vi "Pll_Lock_Detect.vi"(0 "COMPORT":refnum<visa-resource-name>="COM6", 11 "error in (no error)":errorcluster, 12 "CLK_USAGE":u16(ring) items=["EXT CLK", "INT CLK"], 13 "Open Serial":bool, 14 "Close Serial":bool) -> (3 "PllSuccess?(T)":bool, 15 "error out":errorcluster)   [LabVIEW 2018]
panel:
  in  "Command ( ; seperation)":string="pmb 0x69 wr 0xff 00;pmb 0x69 wr 0x07 rd 1"
  out "string":string="caladc\r\n>\ncaladc -r\r\ncaladc delay: 0x00004333\r\n>\r\n"
  out "count?(t)":bool
  out "result(i32)":i32
  out "Reg 0x07":string
  out "Readback Success?(t)":bool
  # "THIS VI IS DESIGNED TO DETECT THE HOLDOVER/LOCK STATE OF  CLOCK"
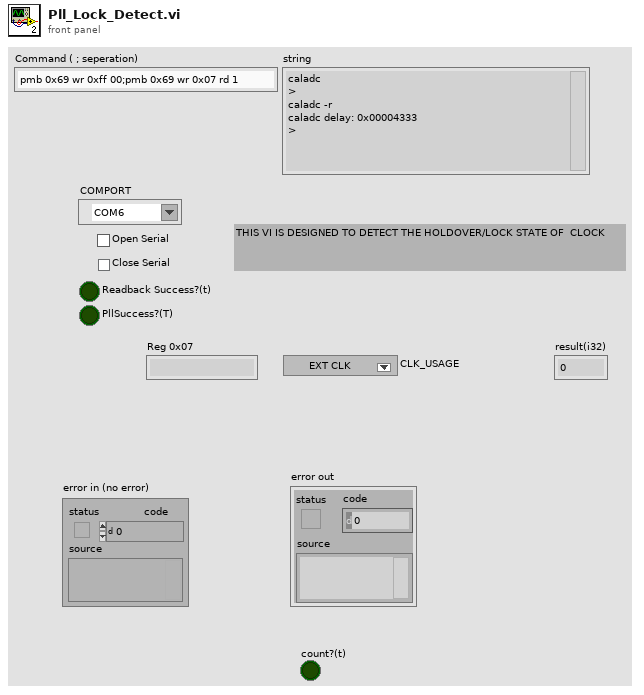
[diagram p1: front panel]
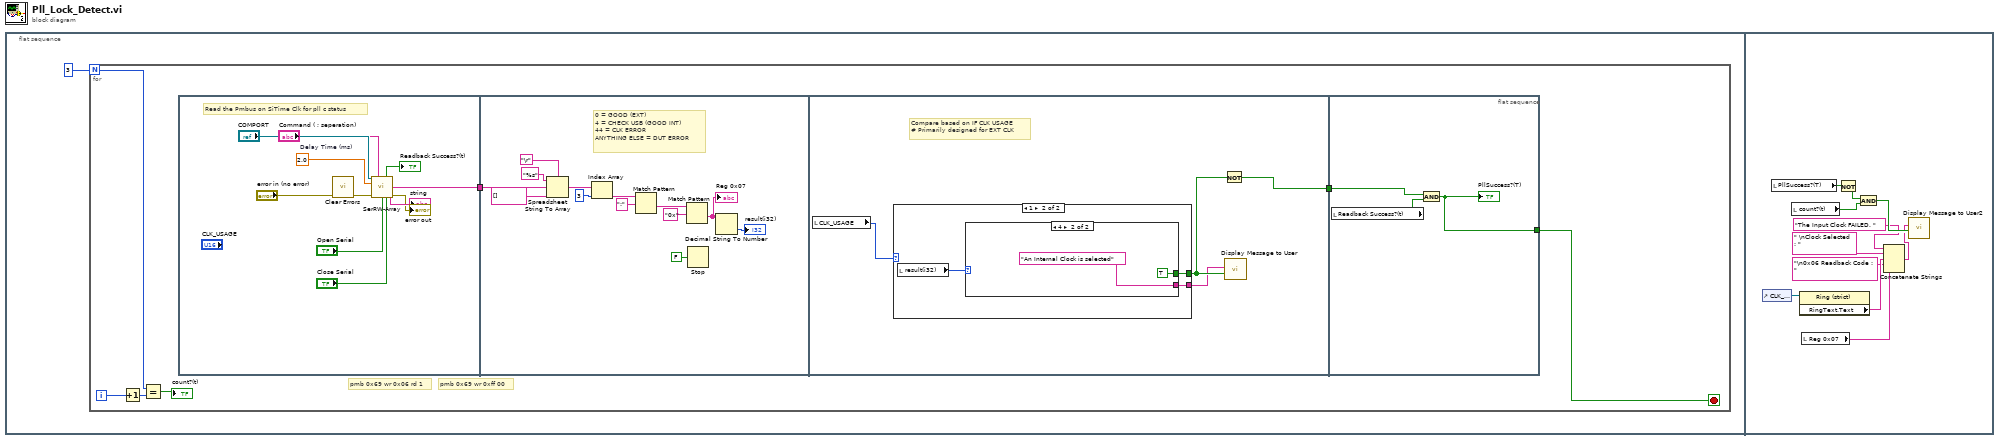
[diagram p0: block diagram]
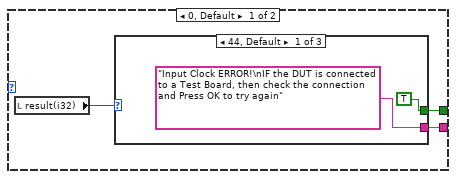
[diagram p2: hidden frame]
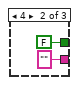
[diagram p3: hidden frame]
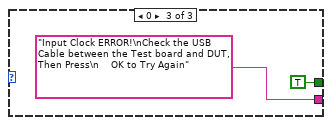
[diagram p4: hidden frame]
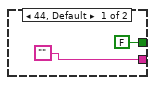
[diagram p5: hidden frame]
diagram:
  n1 = flat-sequence {
    frame #0 {
      n2 = for {
        N: 3 -> [w5]
        i -> [w4]
        stop <- w6 stop-if-true
        # "pmb 0x69 wr 0xff 00"
        # "pmb 0x69 wr 0x06 rd 1"
        n3 = Increment(x=w4) -> (x+1=w3:i32)
        n4 = Equal?(x=w5, y=w3) -> (x = y?=→"count?(t)":bool)
        n5 = flat-sequence {
          tunnel: [w13] -> w8
          tunnel: w8 -> [w22]
          tunnel: [w35] -> w7
          tunnel: w7 -> [w53]
          tunnel: [w52] -> w6
          frame #0 {
            w10 = 2.0  # Delay Time (ms)
            # "Read the Pmbus on SiTime Clk for pll c status"
            n6 = call <vilib>:"Clear Errors.vi"("error in (no error)"="error in (no error)") -> ("error out"=w11:errorcluster)  [unwired: 5 in, 1 out]
            n7 = call "SerRW-Array.vi"("COMPORT"="COMPORT", "Delay Time (ms)"=w10, "error in (no error)"=w11, "Command ( ; seperation)"="Command ( ; seperation)", "Open Serial"="Open Serial", "Close Serial"="Close Serial") -> ("All Success"=→"Readback Success?(t)":bool, "string"=w13:string, "error out"=→"error out":errorcluster)  [unwired: 3 in, 4 out]
            "string" <- w13
          }
          frame #1 {
            # "0 = GOOD (EXT)\n4 = CHECK USB (GOOD INT)\n44 = CLK ERROR\nANYTHING ELSE = DUT ERROR"
            n8 = Spreadsheet String To Array(delimiter (Tab)="\r", format string="%s", spreadsheet string=w22, array type (2D Dbl)=string[] []) -> (array=w27:string[])
            n9 = Index Array(array=w27, index=3) -> (element=w28:string)
            n10 = Match Pattern(string=w28, regular expression=":") -> (after substring=w29:string)  [unwired: 1 in, 3 out]
            n11 = Match Pattern(string=w29, regular expression="0x") -> (after substring=w30:string)  [unwired: 1 in, 3 out]
            "Reg 0x07" <- w30
            n12 = Stop(stop? (T)=FALSE) -> ()
            n13 = Decimal String To Number(string=w30) -> (number=→"result(i32)":i32)  [unwired: 2 in, 1 out]
          }
          frame #2 {
            # "Compare based on IF CLK USAGE\n# Primarily designed for EXT CLK"
            n14 = local read "CLK_USAGE"() -> (w32:u16)
            n15 = case shown="1" w32 {
              tunnel: [w37 w46] -> w34
              tunnel: [w36 w45] -> w33
              frame 0, Default {
                n16 = local read "result(i32)"() -> (w38:i32)
                n17 = case shown="44, Default" w38 {
                  tunnel: [TRUE ("Enable") FALSE ("Enable") TRUE ("Enable")] -> w37
                  tunnel: ["Input Clock ERROR!\nIF the DUT is connected to a Test Board, then check the connection and Press OK to try again" "" "Input Clock ERROR!\nCheck the USB Cable between the Test board and DUT, Then Press\n    OK to Try Again"] -> w36
                  frame 44, Default {
                  }
                  frame 4 {
                  }
                  frame 0 {
                  }
                }
              }
              frame 1 {
                n18 = local read "result(i32)"() -> (w47:i32)
                n19 = case shown="4" w47 {
                  tunnel: [FALSE ("Enable") TRUE ("Enable")] -> w46
                  tunnel: ["" "An Internal Clock is selected"] -> w45
                  frame 44, Default {
                  }
                  frame 4 {
                  }
                }
              }
            }
            n20 = Not(x=w34) -> (.not. x?=w35:bool)
            n21 = call "Display Message to User"("Enable"=w34, "Message"=w33) -> ()  [unwired: 8 in, 2 out]
          }
          frame #3 {
            n22 = local read "Readback Success?(t)"() -> (w54:bool)
            n23 = And(x=w53, y=w54) -> (x .and. y?=w52:bool)
            "PllSuccess?(T)" <- w52
          }
        }
      }
    }
    frame #1 {
      n24 = control-ref of="CLK_USAGE"() -> (w57:refnum<vi>)
      n25 = local read "PllSuccess?(T)"() -> (w65:bool)
      n26 = local read "count?(t)"() -> (w63:bool)
      n27 = property class="Ring (strict)"(reference=w57) -> ("RingText.Text"=w60:string)  [unwired: 1 in, 2 out]
      n28 = local read "Reg 0x07"() -> (w55:string)
      n29 = Not(x=w65) -> (.not. x?=w64:bool)
      n30 = And(x=w64, y=w63) -> (x .and. y?=w62:bool)
      n31 = Concatenate Strings("The Input Clock FAILED. " ("Message"), " \nClock Selected : " ("Message"), w60, "\n0x06 Readback Code : " ("string"), w55) -> (w58:string)
      n32 = call "Display Message to User2"("Enable"=w62, "Message"=w58) -> ()  [unwired: 8 in, 2 out]
    }
  }
